vi "BPM-Chassis03 FPGA.vi"() -> ()   [LabVIEW 2011]
uses:
  <vilib>/rvi/eio/common/nirviEmuTemplateMethod_errors.vi
  <vilib>/eio/EIONode/EIONode.xnode
  <vilib>/eio/EIOMethodNode/EIOMethodNode.xnode
panel:
  out "Timestamp":u32 caption="Tick Count(Ticks)"
  out "Mod1/AI0":fxp<+/-,20,5> format="%.17g"
  out "Mod1/AI2":fxp<+/-,20,5> format="%.17g"
  out "Mod1/AI3":fxp<+/-,20,5> format="%.17g"
  out "Mod2/AI0":fxp<+/-,20,5> format="%.17g"
  out "Mod2/AI1":fxp<+/-,20,5> format="%.17g"
  out "Mod2/AI2":fxp<+/-,20,5> format="%.17g"
  out "Mod2/AI3":fxp<+/-,20,5> format="%.17g"
  out "Mod1/AI1":fxp<+/-,20,5> format="%.17g"
  out "period":u32
  out "delay":u32
  out "dperiod":u32
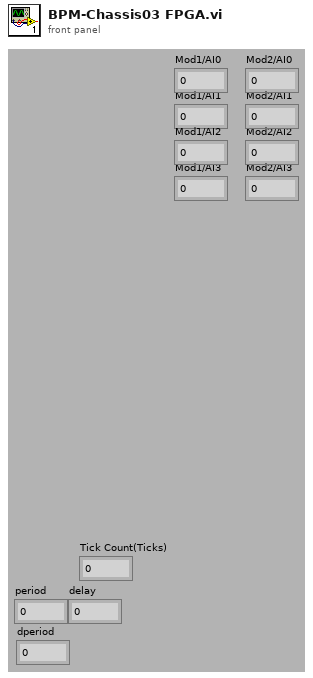
[diagram p1: front panel]
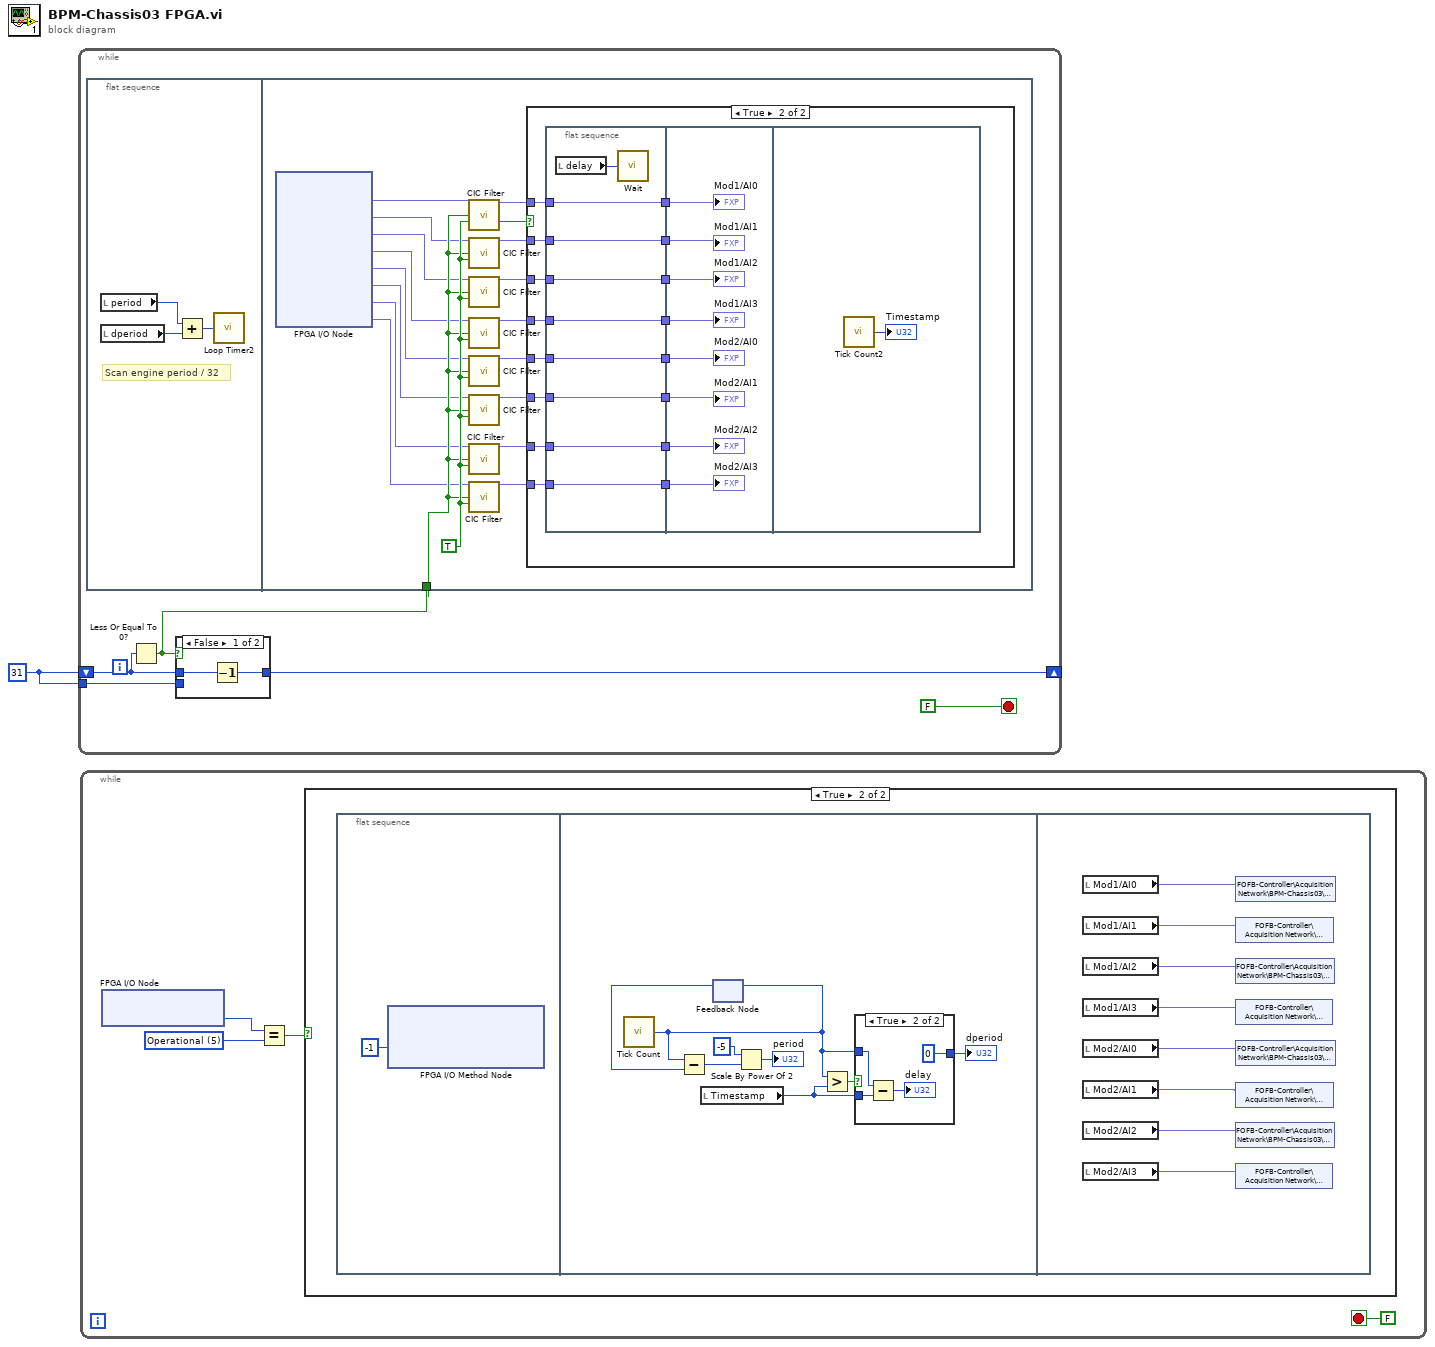
[diagram p0: block diagram]
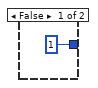
[diagram p5: hidden frame]
diagram:
  w1 = 31
  n1 = while {
    shift-right: [w5] -> _
    shift-left: w1 -> [w4]
    tunnel: w1 -> [w2]
    stop <- FALSE stop-if-true
    n2 = flat-sequence {
      tunnel: w3 -> [w28]
      frame #0 {
        # "Scan engine period / 32"
        n3 = local read "period"() -> (w12:u32)
        n4 = local read "dperiod"() -> (w11:u32)
        n5 = Add(x=w12, y=w11) -> (x+y=w10:u32)
        n6 = call "Loop Timer2"("Count(Ticks)"=w10) -> ()  [unwired: 1 out]
      }
      frame #1 {
        w29 = TRUE ("input valid")
        n7 = xnode "FPGA I/O Node"() -> ("Mod1/AI0"=w20:fxp<+/-,20,5>, "Mod1/AI1"=w19:fxp<+/-,20,5>, "Mod1/AI2"=w18:fxp<+/-,20,5>, "Mod1/AI3"=w17:fxp<+/-,20,5>, "Mod2/AI0"=w16:fxp<+/-,20,5>, "Mod2/AI1"=w15:fxp<+/-,20,5>, "Mod2/AI2"=w14:fxp<+/-,20,5>, "Mod2/AI3"=w13:fxp<+/-,20,5>)  [unwired: 8 in, 8 out]
        n8 = call "CIC Filter.vi"("input data"=w20, "sample"=w28, "input valid"=w29) -> ("output data"=w30:fxp<+/-,20,5>, "output valid"=w31:bool)  [unwired: 10 in, 1 out]
        n9 = call "CIC Filter.vi"("input data"=w19, "sample"=w28, "input valid"=w29) -> ("output data"=w27:fxp<+/-,20,5>)  [unwired: 10 in, 2 out]
        n10 = call "CIC Filter.vi"("input data"=w18, "sample"=w28, "input valid"=w29) -> ("output data"=w26:fxp<+/-,20,5>)  [unwired: 10 in, 2 out]
        n11 = call "CIC Filter.vi"("input data"=w17, "sample"=w28, "input valid"=w29) -> ("output data"=w25:fxp<+/-,20,5>)  [unwired: 10 in, 2 out]
        n12 = call "CIC Filter.vi"("input data"=w16, "sample"=w28, "input valid"=w29) -> ("output data"=w24:fxp<+/-,20,5>)  [unwired: 10 in, 2 out]
        n13 = call "CIC Filter.vi"("input data"=w15, "sample"=w28, "input valid"=w29) -> ("output data"=w23:fxp<+/-,20,5>)  [unwired: 10 in, 2 out]
        n14 = call "CIC Filter.vi"("input data"=w14, "sample"=w28, "input valid"=w29) -> ("output data"=w22:fxp<+/-,20,5>)  [unwired: 10 in, 2 out]
        n15 = call "CIC Filter.vi"("input data"=w13, "sample"=w28, "input valid"=w29) -> ("output data"=w21:fxp<+/-,20,5>)  [unwired: 10 in, 2 out]
        n16 = case shown="True" w31 {
          tunnel: w30 -> [_ w47]
          tunnel: w27 -> [_ w45]
          tunnel: w26 -> [_ w43]
          tunnel: w25 -> [_ w42]
          tunnel: w24 -> [_ w39]
          tunnel: w23 -> [_ w37]
          tunnel: w22 -> [_ w35]
          tunnel: w21 -> [_ w33]
          frame False {
          }
          frame True {
            n17 = flat-sequence {
              tunnel: w47 -> [w56]
              tunnel: [w56] -> w46
              tunnel: w45 -> [w54]
              tunnel: [w54] -> w44
              tunnel: w43 -> [w52]
              tunnel: w42 -> [w53]
              tunnel: [w53] -> w41
              tunnel: [w52] -> w40
              tunnel: w39 -> [w51]
              tunnel: [w51] -> w38
              tunnel: w37 -> [w50]
              tunnel: [w50] -> w36
              tunnel: w35 -> [w49]
              tunnel: [w49] -> w34
              tunnel: w33 -> [w48]
              tunnel: [w48] -> w32
              tunnel: w46 -> [w63]
              tunnel: w44 -> [w64]
              tunnel: w41 -> [w62]
              tunnel: w40 -> [w61]
              tunnel: w38 -> [w60]
              tunnel: w36 -> [w59]
              tunnel: w34 -> [w58]
              tunnel: w32 -> [w57]
              frame #0 {
                n18 = local read "delay"() -> (w55:u32)
                n19 = call "Wait"("Count(Ticks)"=w55) -> ()  [unwired: 1 out]
              }
              frame #1 {
                "Mod1/AI0" <- w63
                "Mod1/AI2" <- w61
                "Mod1/AI3" <- w62
                "Mod2/AI0" <- w60
                "Mod2/AI1" <- w59
                "Mod2/AI2" <- w58
                "Mod2/AI3" <- w57
                "Mod1/AI1" <- w64
              }
              frame #2 {
                n20 = call "Tick Count2"() -> ("Tick Count(Ticks)"=→"Timestamp":u32)
              }
            }
          }
        }
      }
    }
    n21 = Less Or Equal To 0?(x=w4) -> (x <= 0?=w3:bool)
    n22 = case shown="False" w3 {
      tunnel: [w8 w9] -> w5
      tunnel: w4 -> [w7 _]
      tunnel: w2 -> [_ w9]
      frame False {
        n23 = Decrement(x=w7) -> (x-1=w8:i32)
      }
      frame True {
      }
    }
  }
  n24 = while {
    stop <- FALSE stop-if-true
    w68 = u8 5 items=["Init"=1, "PreOp"=2, "Bootstrap"=3, "SafeOp"=4, "Operational"=5]
    n25 = xnode "FPGA I/O Node"() -> ("EtherCAT State"=w67:u8)  [unwired: 1 in, 1 out]
    n26 = Equal?(x=w67, y=w68) -> (x = y?=w66:bool)
    n27 = case shown="True" w66 {
      frame False {
      }
      frame True {
        n28 = flat-sequence {
          frame #0 {
            n29 = xnode "FPGA I/O Method Node"("Timeout"=-1) -> ()  [unwired: 1 in, 2 out]
          }
          frame #1 {
            n30 = call "Tick Count"() -> ("Tick Count(Ticks)"=w72:u32)
            n31 = local read "Timestamp"() -> (w74:u32)
            n32 = feedback #1() -> (w71:u32)  [unwired: 1 in]
            n33 = Subtract(x=w72, y=w71) -> (x-y=w77:u32)
            n34 = feedback-in #1(w72) -> ()
            n35 = Scale By Power Of 2(n=i8 -5, x=w77) -> (x*2^n=→"period":u32)
            n36 = Greater?(x=w72, y=w74) -> (0:w75:bool)
            n37 = case shown="True" w75 {
              tunnel: w72 -> [_ w83]
              tunnel: w74 -> [_ w82]
              tunnel: [u32 1 ("dt 2") u32 0 ("dt 2")] -> w73
              frame False {
              }
              frame True {
                n38 = Subtract(x=w83, y=w82) -> (x-y=→"delay":u32)
              }
            }
            "dperiod" <- w73
          }
          frame #2 {
            n39 = local read "Mod1/AI0"() -> (w91:fxp<+/-,20,5>)
            n40 = local read "Mod1/AI1"() -> (w90:fxp<+/-,20,5>)
            n41 = local read "Mod1/AI2"() -> (w89:fxp<+/-,20,5>)
            n42 = local read "Mod1/AI3"() -> (w88:fxp<+/-,20,5>)
            n43 = local read "Mod2/AI0"() -> (w87:fxp<+/-,20,5>)
            n44 = local read "Mod2/AI1"() -> (w86:fxp<+/-,20,5>)
            n45 = local read "Mod2/AI2"() -> (w85:fxp<+/-,20,5>)
            n46 = local read "Mod2/AI3"() -> (w84:fxp<+/-,20,5>)
            n47 = shared-variable "FOFB-Controller\\Acquisition Network\\BPM-Chassis03\\User-Defined Variables\\AMP06AH"(w91) -> ()  [unwired: 1 in, 1 out]
            n48 = shared-variable "FOFB-Controller\\Acquisition Network\\BPM-Chassis03\\User-Defined Variables\\AMP06AV"(w90) -> ()  [unwired: 1 in, 1 out]
            n49 = shared-variable "FOFB-Controller\\Acquisition Network\\BPM-Chassis03\\User-Defined Variables\\AMP06BH"(w89) -> ()  [unwired: 1 in, 1 out]
            n50 = shared-variable "FOFB-Controller\\Acquisition Network\\BPM-Chassis03\\User-Defined Variables\\AMP06BV"(w88) -> ()  [unwired: 1 in, 1 out]
            n51 = shared-variable "FOFB-Controller\\Acquisition Network\\BPM-Chassis03\\User-Defined Variables\\AMP07AH"(w87) -> ()  [unwired: 1 in, 1 out]
            n52 = shared-variable "FOFB-Controller\\Acquisition Network\\BPM-Chassis03\\User-Defined Variables\\AMP07AV"(w86) -> ()  [unwired: 1 in, 1 out]
            n53 = shared-variable "FOFB-Controller\\Acquisition Network\\BPM-Chassis03\\User-Defined Variables\\AMP07BH"(w85) -> ()  [unwired: 1 in, 1 out]
            n54 = shared-variable "FOFB-Controller\\Acquisition Network\\BPM-Chassis03\\User-Defined Variables\\AMP07BV"(w84) -> ()  [unwired: 1 in, 1 out]
          }
        }
      }
    }
  }
